vi "4461 - Create Reference Waveforms.vi"(6 "sampling info":cluster{"Fs":dbl, "#s":dbl}={"Fs"=1000.0, "#s"=1000.0} {"Fs" format="%.2p"}, 8 "error in (no error)":errorcluster, 10 "reset signal":bool, 11 "Lockin":T1={"REF f (Hz)"=[13.0, 13.0, 13.0, 13.0, 13.0, 13.0, 13.0, 13.0], "REF phi (°)"=[0.0, 0.0, 0.0, 0.0, 0.0, 0.0, 0.0, 0.0]} {"REF phi (°)" format="%#_3g"}) -> (0 "error out":errorcluster, 1 "phase out":dbl[](array[numeric]), 2 "AO Array":waveform(dbl)[](array[waveform]), 3 "Lockin 2":T1={"REF f (Hz)"=[13.0, 13.0, 13.0, 13.0, 13.0, 13.0, 13.0, 13.0], "REF phi (°)"=[0.0, 0.0, 0.0, 0.0, 0.0, 0.0, 0.0, 0.0]} {"REF phi (°)" format="%#_3g"})   [LabVIEW 2016]
uses:
  Typedefs/REF-cluster.ctl
  Typedefs/REF_f-array.ctl
  Typedefs/REF_phi-array.ctl
  <vilib>/measure/NI_MABase.lvlib
panel:
  out "Waveform Graph 2":waveform(dbl)[](graph)
  out "Numeric":i32
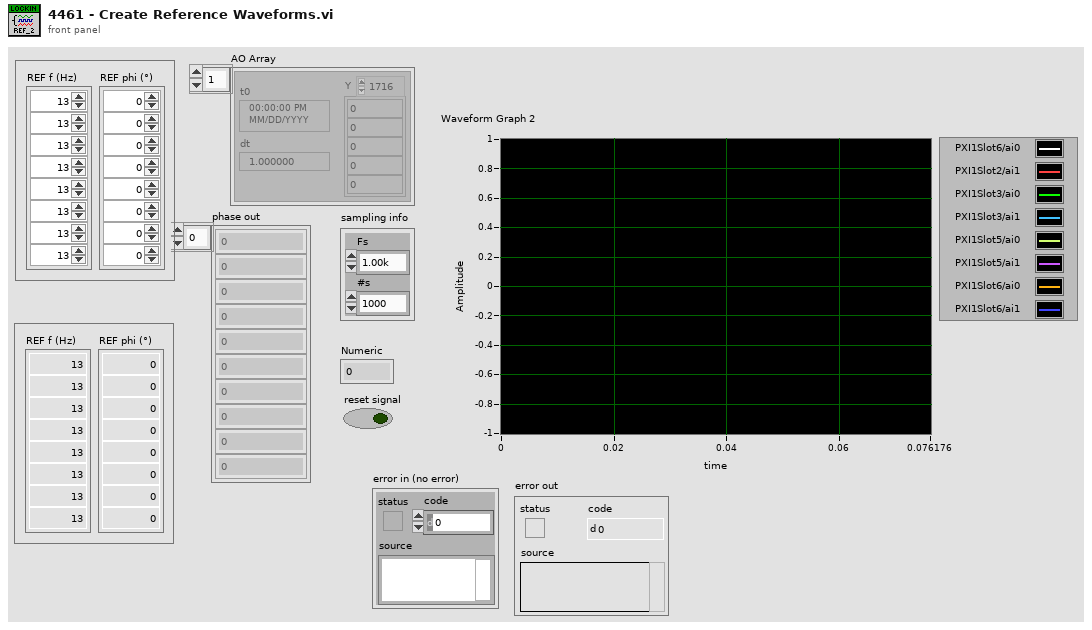
[diagram p1: front panel]
types:
  T1 = typedef "REF-cluster.ctl" = cluster{"REF f (Hz)":T2, "REF phi (°)":T3}
  T2 = typedef "REF_f-array.ctl" = dbl[]
  T3 = typedef "REF_phi-array.ctl" = dbl[]
  T4 = enum16{"Sine Wave", "Triangle Wave", "Square Wave", "Sawtooth Wave"}
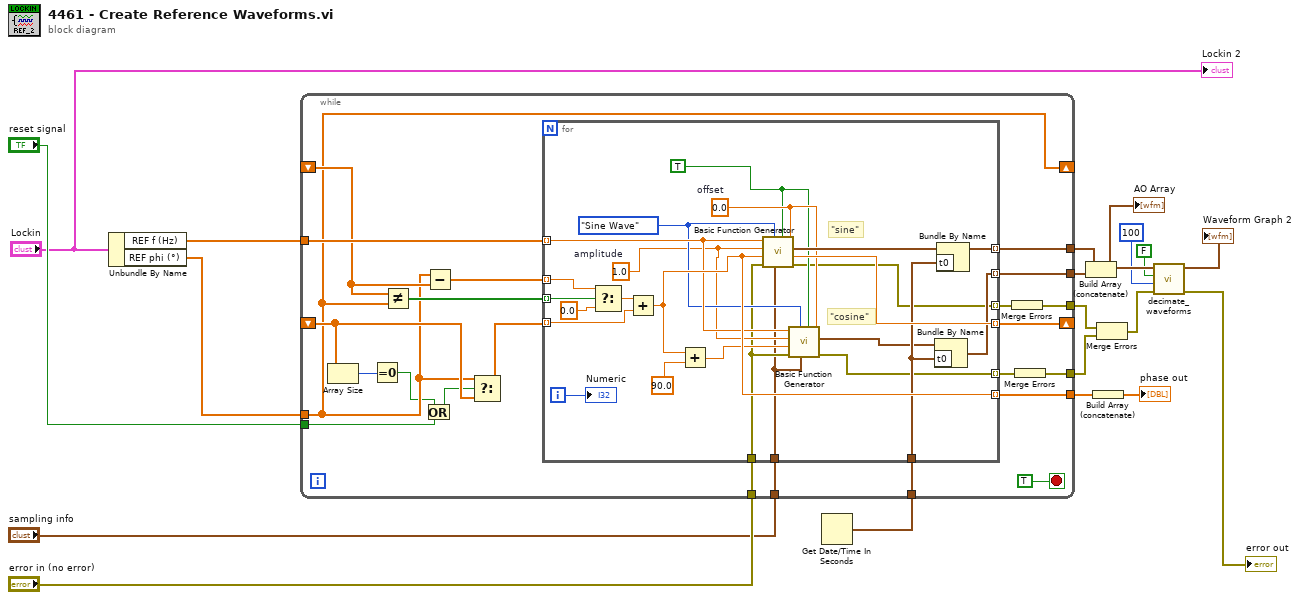
[diagram p0: block diagram]
diagram:
  n1 = Unbundle By Name("Lockin") -> ("REF f (Hz)"=w14:T2, "REF phi (°)"=w4:T3)
  n2 = Get Date/Time In Seconds() -> (seconds since 1Jan1904=w5:timestamp)
  n3 = while {
    tunnel: "sampling info" -> [w42]
    tunnel: [w41] -> w15
    tunnel: w4 -> [w30]
    tunnel: w14 -> [w40]
    shift-right: [w30] -> _
    shift-left: _ -> [w37]
    shift-right: [w35] -> _
    shift-left: _ -> [w32]
    tunnel: w5 -> [w33]
    tunnel: "reset signal" -> [w27]
    tunnel: [w26] -> w18
    tunnel: [w25] -> w16
    tunnel: "error in (no error)" -> [w24]
    tunnel: [w22] -> w8
    tunnel: [w20] -> w9
    stop <- TRUE stop-if-true
    n4 = Array Size(array=w32) -> (size(s)=w31:i32)
    n5 = Equal To 0?(x=w31) -> (x = 0?=w28:bool)
    n6 = Not Equal?(x=w37, y=w30) -> (x != y?=w38:bool[])
    n7 = Or(x=w28, y=w27) -> (x .or. y?=w29:bool)
    n8 = Subtract(x=w30, y=w37) -> (x-y=w36:T3)
    n9 = Select(t=w30, s=w29, f=w32) -> (s? t:f=w34:T3)
    n10 = for {
      tunnel: w40 -> [w54] mode=indexing
      tunnel: [w65] -> w41 mode=indexing
      tunnel: w42 -> [w45]
      tunnel: w38 -> [w59] mode=indexing
      tunnel: w36 -> [w61] mode=indexing
      tunnel: [w57] -> w35 mode=indexing
      tunnel: w34 -> [w62] mode=indexing
      tunnel: w33 -> [w53]
      tunnel: [w56] -> w26 mode=indexing
      tunnel: [w51] -> w25 mode=indexing
      tunnel: w24 -> [w46]
      tunnel: [w44] -> w23 mode=indexing
      tunnel: [w43] -> w21 mode=indexing
      i -> [w58]
      w47 = TRUE ("reset signal")
      w49 = 0.0  # offset
      w50 = T4."Sine Wave" ("signal type")
      w48 = 1.0  # amplitude
      # "\"cosine\""
      # "\"sine\""
      n11 = Select(t=w61, s=w59, f=0.0) -> (s? t:f=w63:dbl)
      n12 = Add(x=w63, y=w62) -> (x+y=w56:dbl)
      n13 = Add(x=w56, y=90.0) -> (x+y=w55:dbl)
      n14 = call <vilib>:"Basic Function Generator.vi"("offset"=w49, "reset signal"=w47, "sampling info"=w45, "signal type"=w50, "error in (no error)"=w46, "phase"=w56, "amplitude"=w48, "frequency"=w54) -> ("error out"=w44:errorcluster, "phase out"=w57:dbl, "signal out"=w66:waveform(dbl))  [unwired: 1 in]
      n15 = call <vilib>:"Basic Function Generator.vi"("offset"=w49, "reset signal"=w47, "sampling info"=w45, "signal type"=w50, "error in (no error)"=w46, "phase"=w55, "amplitude"=w48, "frequency"=w54) -> ("error out"=w43:errorcluster, "signal out"=w52:waveform(dbl))  [unwired: 1 in, 1 out]
      n16 = Bundle By Name(cluster=w52, "t0"=w53) -> (w51:waveform(dbl))
      n17 = Bundle By Name(cluster=w66, "t0"=w53) -> (w65:waveform(dbl))
      "Numeric" <- w58
    }
    n18 = Merge Errors(w23) -> (w22:errorcluster)
    n19 = Merge Errors(w21) -> (w20:errorcluster)
  }
  n20 = Build Array (concatenate)(w15, w16) -> (w11:waveform(dbl)[])
  "AO Array" <- w11
  n21 = Build Array (concatenate)(w18) -> (→"phase out":dbl[])
  n22 = Merge Errors(w8, w9) -> (w7:errorcluster)
  n23 = call "decimate_waveforms.vi"("Input Signal"=w11, "averaging"=FALSE, "decimating factor"=100, "error in (no error)"=w7) -> ("Decimated Waveforms"=→"Waveform Graph 2":waveform(dbl)[], "error out"=→"error out":errorcluster)  [unwired: 5 in]
  "Lockin 2" <- "Lockin"
